vi "FT conversion.vi"(2 "Control Box":T1={"Force Divider"=50.0, "Torque Divider"=2000.0}, 3 "Raw Data":u16[](array[numeric]), 4 "Bias":dbl[](array[numeric])=[0.0, 0.0, 0.0, 0.0, 0.0, 0.0]) -> (0 "ForceTorque":dbl[](array[numeric]), 1 "Unbiased DATA":dbl[](array[numeric]))   [LabVIEW 2011]
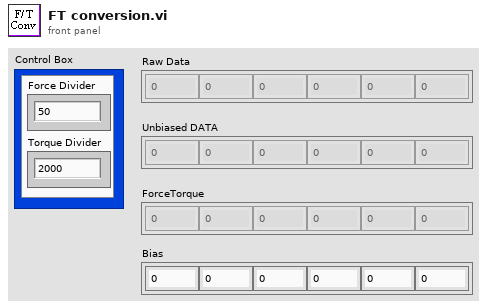
[diagram p1: front panel]
types:
  T1 = cluster{"Force Divider":dbl, "Torque Divider":dbl}
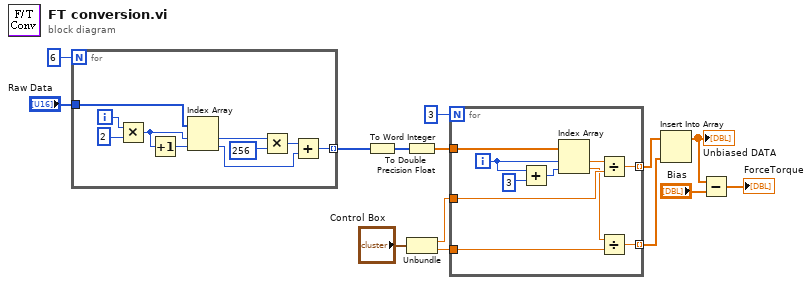
[diagram p0: block diagram]
diagram:
  n1 = for {
    N: 6 -> [_]
    tunnel: "Raw Data" -> [w20]
    tunnel: [w15] -> w8 mode=indexing
    i -> [w24]
    n2 = Multiply(x=w24, y=2) -> (x*y=w21:i32)
    n3 = Increment(x=w21) -> (x+1=w22:i32)
    n4 = Index Array(array=w20, index #1=w21, index #2=w22) -> (element #1=w19:u16, element #2=w17:u16)
    n5 = Multiply(x=w19, y=256) -> (x*y=w16:i32)
    n6 = Add(x=w16, y=w17) -> (x+y=w15:i32)
  }
  n7 = To Word Integer(number=w8) -> (16bit integer=w13:i16[])
  n8 = To Double Precision Float(number=w13) -> (double precision float=w6:dbl[])
  n9 = Unbundle("Control Box") -> ("Force Divider"=w5:dbl, "Torque Divider"=w4:dbl)
  n10 = for {
    N: 3 -> [_]
    tunnel: w6 -> [w34]
    tunnel: w5 -> [w29]
    tunnel: w4 -> [w27]
    tunnel: [w26] -> w3 mode=indexing
    tunnel: [w25] -> w2 mode=indexing
    i -> [w30]
    n11 = Add(x=w30, y=3) -> (x+y=w31:i32)
    n12 = Index Array(array=w34, index #1=w30, index #2=w31) -> (element #1=w32:dbl, element #2=w28:dbl)
    n13 = Divide(x=w32, y=w29) -> (x/y=w26:dbl)
    n14 = Divide(x=w28, y=w27) -> (x/y=w25:dbl)
  }
  n15 = Insert Into Array(array=w3, new element=w2) -> (w1:dbl[])  [unwired: 1 in]
  "Unbiased DATA" <- w1
  n16 = Subtract(x=w1, y="Bias") -> (x-y=→"ForceTorque":dbl[])
